vi "fpga_128ch-Scheduler.vi"() -> (0 "FIFO Schedule":u8, 1 "Main clock":u32)   [LabVIEW 2011]
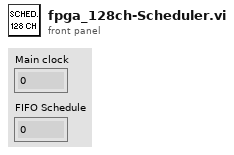
[diagram p1: front panel]
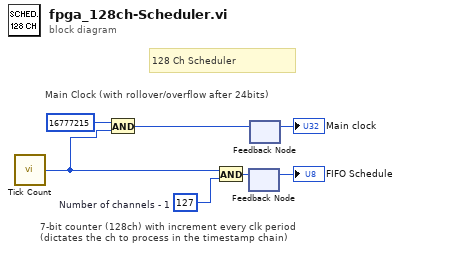
[diagram p0: block diagram]
diagram:
  w7 = u32 127  # Number of channels - 1
  # "128 Ch Scheduler"
  # "Main Clock (with rollover/overflow after 24bits)"
  # "7-bit counter (128ch) with increment every clk period\n(dictates the ch to process in the timestamp chain)"
  n1 = call "Tick Count"() -> ("Tick Count(Ticks)"=w1:u32)
  n2 = And(x=u32 16777215, y=w1) -> (x .and. y?=w5:u32)
  n3 = And(x=w1, y=w7) -> (x .and. y?=w6:u32)
  n4 = feedback-in #1(w6) -> ()
  n5 = feedback #1() -> (→"FIFO Schedule":u32)  [unwired: 1 in]
  n6 = feedback-in #2(w5) -> ()
  n7 = feedback #2() -> (→"Main clock":u32)  [unwired: 1 in]
